vi "Build Voltage Scaling RT Data.vi"(6 "Custom Device Ref":T2 format="%.0x", 8 "error in (no error)":errorcluster, 9 "DataReplayVoltages in":T3[](array[typedef]), 10 "DataReplay":T1, 11 "Replay ref in":T2 format="%.0x") -> (0 "error out":errorcluster, 1 "DataReplayVoltages out":T3[](array[typedef]), 2 "DataReplay dup":T1, 3 "Replay ref dup":T2 format="%.0x")   [LabVIEW 2011, in "Engine Sim System Explorer.lvlib"]
uses:
  Engine Sim System Explorer.lvlib
  Shared/DataReplayVoltageConfig.ctl
  Shared/DataReplayConfig.ctl
  <vilib>/NI Veristand/Custom Device API/Custom Device Item Ref.ctl
  Shared/Engine Simulation Global.vi
  <vilib>/NI Veristand/Custom Device API/Get Item Property (Boolean).vi
  <vilib>/NI Veristand/Custom Device Tools/Custom Device Utility Library/NI VeriStand - Search for Item by Name.vi
  <vilib>/NI Veristand/Custom Device API/Custom Device API.lvlib
  Engine Simulation Shared.lvlib
  <vilib>/NI Veristand/Custom Device Tools/Custom Device Utility Library/Custom Device Utility Library.lvlib
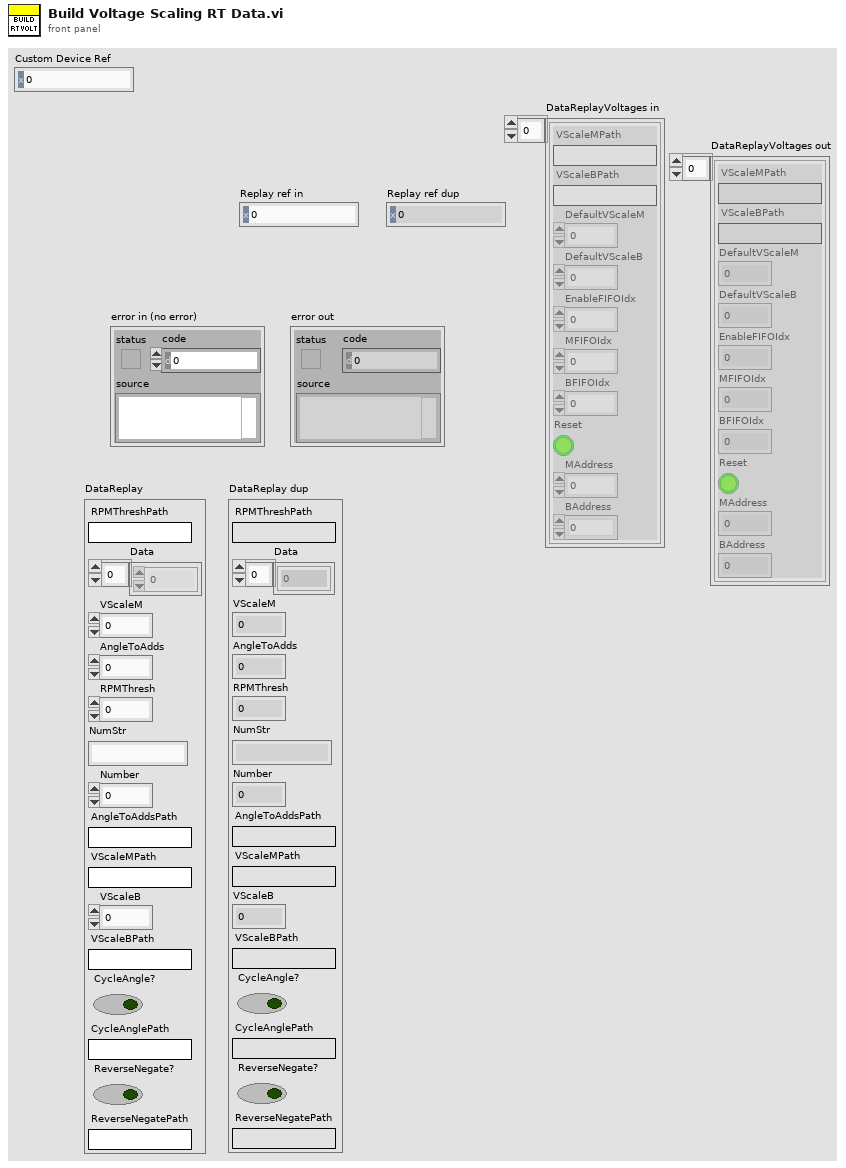
[diagram p1: front panel]
types:
  T1 = typedef "Engine Simulation Shared.lvlib/DataReplayConfig.ctl" = cluster{"RPMThreshPath":string, "Data":i16[], "VScaleM":u32, "AngleToAdds":u32, "RPMThresh":u64, "NumStr":string, "Number":i8, "AngleToAddsPath":string, "VScaleMPath":string, "VScaleB":i32, "VScaleBPath":string, "CycleAngle?":bool, "CycleAnglePath":string, "ReverseNegate?":bool, "ReverseNegatePath":string}
  T2 = typedef "Custom Device API.lvlib/Custom Device Item Ref.ctl" = u64
  T3 = typedef "Engine Simulation Shared.lvlib/DataReplayVoltageConfig.ctl" = cluster{"VScaleMPath":string, "VScaleBPath":string, "DefaultVScaleM":u32, "DefaultVScaleB":i32, "EnableFIFOIdx":i32, "MFIFOIdx":i32, "BFIFOIdx":i32, "Reset":bool, "MAddress":u32, "BAddress":u32}
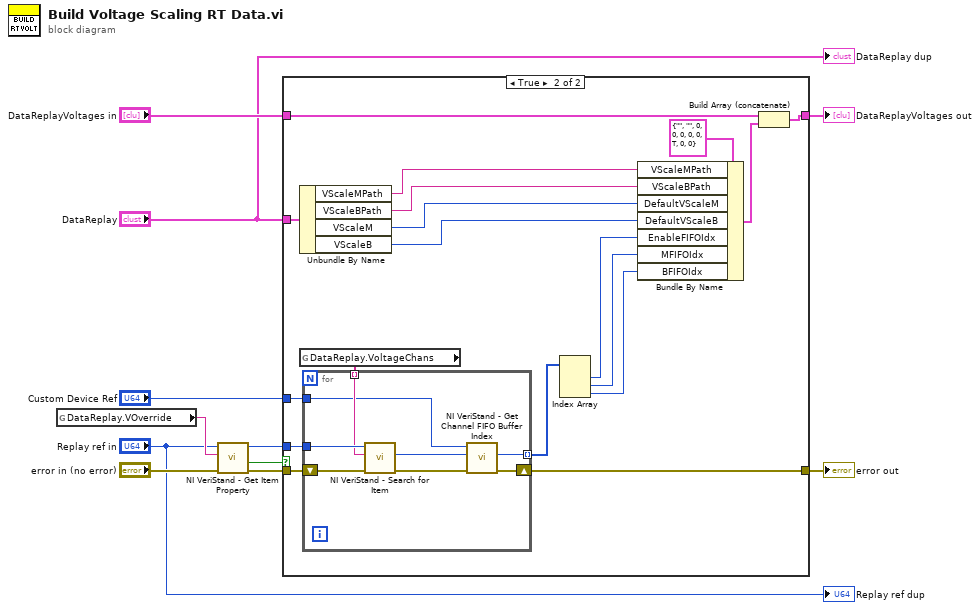
[diagram p0: block diagram]
diagram:
  n1 = global read "Engine Simulation Global.vi" "DataReplay.VOverride"() -> (w10:string)
  n2 = call-poly <vilib>:"NI VeriStand - Get Item Property.vi"("error in (no error)"="error in (no error)", "Property Name"=w10, "Item Ref in"="Replay ref in") -> ("error out"=w6:errorcluster, "Value"=w9:bool, "Item Ref out"=w5:T2)  [unwired: 5 in, 1 out]
  n3 = case shown="True" w9 {
    tunnel: [w13 w30] -> w8
    tunnel: "DataReplayVoltages in" -> [w13 w31]
    tunnel: "DataReplay" -> [_ w29]
    tunnel: w6 -> [w12 w22]
    tunnel: w5 -> [_ w21]
    tunnel: "Custom Device Ref" -> [_ w19]
    tunnel: [w12 w14] -> w3
    frame False {
    }
    frame True {
      n4 = Unbundle By Name(w29) -> ("VScaleMPath"=w26:string, "VScaleBPath"=w25:string, "VScaleM"=w24:u32, "VScaleB"=w23:i32)
      n5 = global read "Engine Simulation Global.vi" "DataReplay.VoltageChans"() -> (w20:string[])
      n6 = for {
        tunnel: w21 -> [w38]
        shift-right: [w33] -> w14
        shift-left: w22 -> [w39]
        tunnel: w20 -> [w37] mode=indexing
        tunnel: w19 -> [w34]
        tunnel: [w32] -> w18 mode=indexing
        n7 = call-poly <vilib>:"NI VeriStand - Search for Item.vi"("error in"=w39, "Item Name"=w37, "Section Ref in"=w38) -> ("error out"=w36:errorcluster, "Item Ref"=w35:T2)  [unwired: 5 in, 2 out]
        n8 = call <vilib>:"NI VeriStand - Get Channel FIFO Buffer Index.vi"("error in"=w36, "Channel Ref"=w35, "Device Ref in"=w34) -> ("error out"=w33:errorcluster, "Channel FIFO Buffer Index"=w32:i32)  [unwired: 4 in, 3 out]
      }
      n9 = Index Array(array=w18) -> (element #1=w17:i32, element #2=w16:i32, element #3=w15:i32)  [unwired: 3 in]
      n10 = Bundle By Name(cluster=T3 {"VScaleMPath"="", "VScaleBPath"="", "DefaultVScaleM"=0, "DefaultVScaleB"=0, "EnableFIFOIdx"=0, "MFIFOIdx"=0, "BFIFOIdx"=0, "Reset"=TRUE, "MAddress"=0, "BAddress"=0} ("Profile Config"), "VScaleMPath"=w26, "VScaleBPath"=w25, "DefaultVScaleM"=w24, "DefaultVScaleB"=w23, "EnableFIFOIdx"=w17, "MFIFOIdx"=w16, "BFIFOIdx"=w15) -> (w27:T3)
      n11 = Build Array (concatenate)(w31, w27) -> (w30:T3[])
    }
  }
  "error out" <- w3
  "DataReplayVoltages out" <- w8
  "Replay ref dup" <- "Replay ref in"
  "DataReplay dup" <- "DataReplay"
